vi "Process Pupil or Cornea ReflectionPerc.vi"(0 "Image In":T1, 1 "ROI":i32[](array[numeric]), 3 "Threshold":u8=130, 4 "Direction to keep":enum16{"Above", "Below"}(ring)=enum."Below", 5 "error in (no error)":errorcluster, 6 "Display":bool, 7 "Fit type":enum16{"Circle", "Ellipse"}(ring)=enum."Ellipse", 9 "Subsampling":i32=1, 10 "Color":u32(colorbox)=16711680, 11 "use % thresh":bool, 12 "Display Overlay":bool, 13 "Points to show":enum16{"All points", "Fit points"}(ring)) -> (14 "Image out":T1, 15 "x position":dbl, 17 "y position":dbl, 18 "diameter":dbl, 19 "error out":errorcluster)   [LabVIEW 2013]
uses:
  <vilib>/vision/Image Controls.llb/IMAQ Image.ctl
  Outline/Outline.lvclass
  <vilib>/Analysis/baseanly.llb/Mean (DBL).vi
  <vilib>/vision/NI_Vision_Development_Module.lvlib
  <vilib>/Analysis/NI_AALBase.lvlib
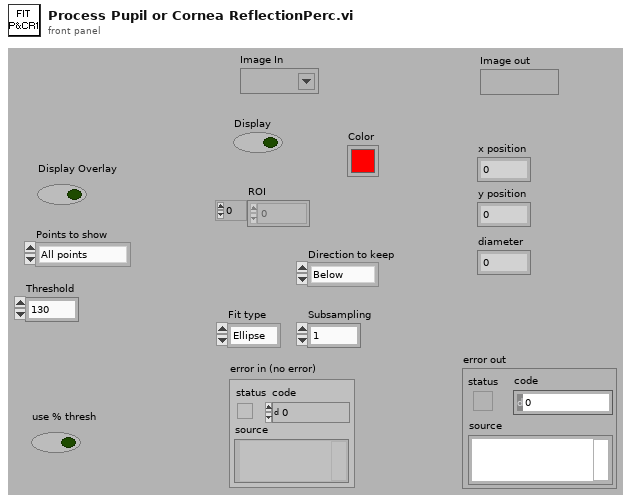
[diagram p1: front panel]
types:
  T1 = typedef "IMAQ Image.ctl" = refnum<image>
  T2 = cluster{"ROI[0]":i32, "ROI[1]":i32, "ROI[2]":i32, "ROI[3]":i32}
  T3 = cluster{"Center":cluster{"X":sgl, "Y":sgl}, "Radius":dbl}
  T4 = cluster{"Center":cluster{"X":sgl, "Y":sgl}, "Major Axis":cluster{"Point 1":cluster{"X":sgl, "Y":sgl}, "Point 2":cluster{"X":sgl, "Y":sgl}}, "Minor Axis":cluster{"Point 1":cluster{"X":sgl, "Y":sgl}, "Point 2":cluster{"X":sgl, "Y":sgl}}}
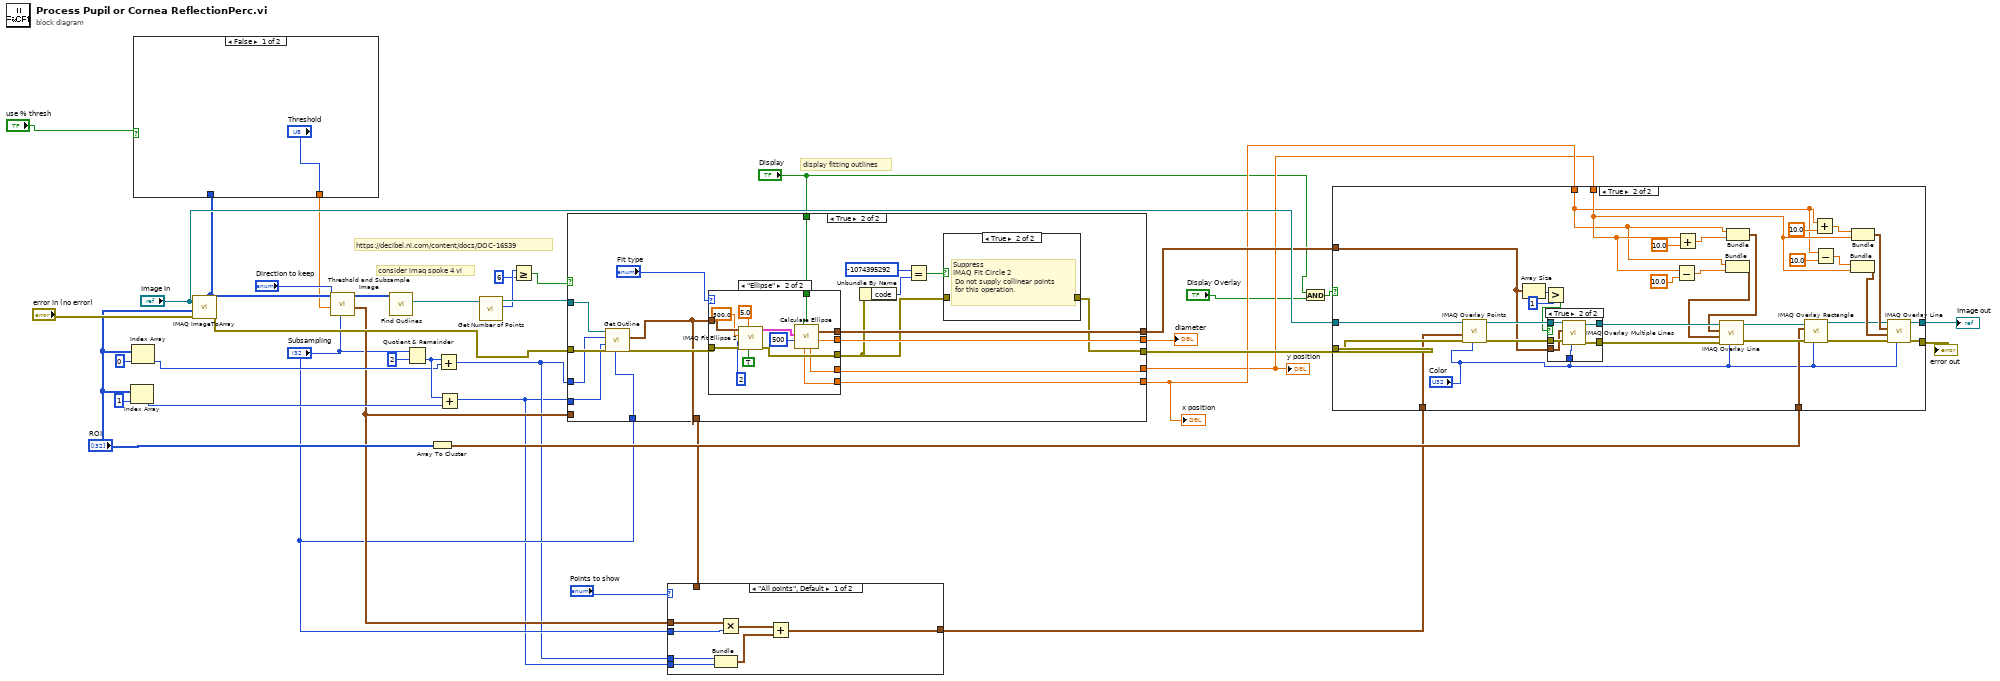
[diagram p0: block diagram]
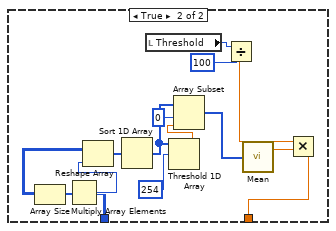
[diagram p2: hidden frame]
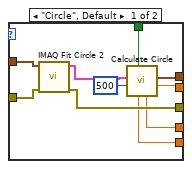
[diagram p8: hidden frame]
diagram:
  # "https://decibel.ni.com/content/docs/DOC-16539"
  # "consider imaq spoke 4 vi"
  # "display fitting outlines"
  n1 = Index Array(array="ROI", index=1) -> (element=w30:i32)
  n2 = Index Array(array="ROI", index=0) -> (element=w33:i32)
  n3 = call "IMAQ ImageToArray"("error in (no error)"="error in (no error)", "Optional Rectangle"="ROI", "Image"="Image In") -> ("error out"=w24:errorcluster, "Image Pixels (U8)"=w3:u8[][])  [unwired: 1 in, 3 out]
  n4 = case shown="False" "use % thresh" {
    tunnel: w3 -> [_ w51]
    tunnel: ["Threshold" w49] -> w1
    frame False {
    }
    frame True {
      n5 = Array Size(array=w51) -> (size(s)=w52:i32[])
      n6 = Multiply Array Elements(1:w52) -> (0:w53:i32)
      n7 = Reshape Array(w51, w53) -> (w45:u8[])
      n8 = Sort 1D Array(array=w45) -> (sorted array=w43:u8[])
      n9 = local read "Threshold"() -> (w48:u8)
      n10 = Threshold 1D Array(2:i16 254 ("threshold y"), 3:w43) -> (0:w42:dbl)  [unwired: 1 in]
      n11 = Array Subset(array=w43, index=0, length=w42) -> (w40:u8[])
      n12 = Divide(x=w48, y=u8 100) -> (x/y=w47:dbl)
      n13 = call-poly <vilib>:"Mean.vi"("X"=w40) -> ("mean"=w50:dbl)  [unwired: 1 out]
      n14 = Multiply(x=w47, y=w50) -> (x*y=w49:dbl)
    }
  }
  n15 = call "Threshold and Subsample Image.vi"("Subsample"="Subsampling", "Threshold"=w1, "Direction to keep"="Direction to keep", "Image Pixels (U8)"=w3) -> ("Cross Threshold Points"=w12:cluster{"X":i32, "Y":i32}[], "Image Pixels (U8) out"=w37:u8[][])  [unwired: 6 in]
  n16 = call "Find Outlines.vi"("Image Pixels (U8)"=w37) -> ("Largest Outline"=w25:refnum<class "Outline.lvclass">)  [unwired: 9 in, 1 out]
  n17 = Quotient & Remainder(x="Subsampling", y=2) -> (floor(x/y)=w35:i32)  [unwired: 1 out]
  n18 = Array To Cluster(array="ROI") -> (cluster=w20:T2)
  n19 = Add(x=w35, y=w33) -> (x+y=w9:i32)
  n20 = Add(x=w35, y=w30) -> (x+y=w8:i32)
  n21 = call-dynamic "Get Number of Points.vi"("Outline in"=w25) -> ("Number of points"=w28:i32, "Outline out"=w29:refnum<class "Outline.lvclass">)  [unwired: 8 in, 1 out]
  n22 = Greater Or Equal?(x=w28, y=6) -> (x >= y?=w26:bool)
  n23 = case shown="True" w26 {
    tunnel: w24 -> [w54 w72]
    tunnel: [w54 w60] -> w23
    tunnel: w9 -> [_ w57]
    tunnel: w8 -> [_ w56]
    tunnel: w29 -> [_ w71]
    tunnel: "Subsampling" -> [_ w58]
    tunnel: [_ w69] -> w19
    tunnel: [_ w67] -> w18
    tunnel: [_ w66] -> w17
    tunnel: [_ w65] -> w14
    tunnel: "Display" -> [_ w59]
    tunnel: w12 -> [_ _]
    tunnel: [_ w55] -> w13
    frame False {
    }
    frame True {
      n24 = call-dynamic "Get Outline.vi"("Scale Factor"=w58, "error in (no error)"=w72, "Y Offset"=w56, "X Offset"=w57, "Outline in"=w71) -> ("error out"=w68:errorcluster, "Outline"=w55:cluster{"X":i32, "Y":i32}[])  [unwired: 4 in, 1 out]
      n25 = case shown="\"Ellipse\"" "Fit type" {
        tunnel: w68 -> [w82 w97]
        tunnel: w55 -> [w83 w96]
        tunnel: [w81 w95] -> w61
        tunnel: [w79 w93] -> w69
        tunnel: [w78 w88] -> w67
        tunnel: [w77 w87] -> w66
        tunnel: [w75 w85] -> w65
        tunnel: w59 -> [w74 w84]
        frame "Circle", Default {
          n26 = call "IMAQ Fit Circle 2"("error in (no error)"=w82, "Radial Points"=w83) -> ("error out"=w81:errorcluster, "Circle"=w80:T3)  [unwired: 4 in, 4 out]
          n27 = call "Calculate Circle.vi"("Display"=w74, "steps"=500, "Circle"=w80) -> ("Diameter"=w75:dbl, "Circle Coordinates"=w79:cluster{"X":i32, "Y":i32}[], "y position"=w77:dbl, "x position"=w78:dbl)  [unwired: 5 in]
        }
        frame "Ellipse" {
          n28 = call "IMAQ Fit Ellipse 2"("Reject Outliers (FALSE)"=TRUE, "Pixel Radius"=5.0, "error in (no error)"=w97, "Maximum Iterations"=2, "Minimum Score"=500.0, "Radial Points"=w96) -> ("error out"=w95:errorcluster, "Ellipse"=w92:T4)  [unwired: 4 out]
          n29 = call "Calculate Ellipse.vi"("Display"=w84, "steps"=500, "Ellipse"=w92) -> ("Effective Diameter"=w85:sgl, "Ellipse Coordinates"=w93:cluster{"X":i32, "Y":i32}[], "y position"=w87:dbl, "x position"=w88:dbl)  [unwired: 5 in]
        }
      }
      n30 = Unbundle By Name(w61) -> ("code"=w64:i32)
      n31 = Equal?(x=-1074395292, y=w64) -> (x = y?=w62:bool)
      n32 = case shown="True" w62 {
        tunnel: w61 -> [w73 _]
        tunnel: [w73 _] -> w60
        frame False {
        }
        frame True {
          # "Suppress\nIMAQ Fit Circle 2\n Do not supply collinear points\n for this operation."
        }
      }
    }
  }
  "diameter" <- w14
  "x position" <- w18
  "y position" <- w17
  n33 = case shown="\"All points\", Default" "Points to show" {
    tunnel: w12 -> [w102 _]
    tunnel: "Subsampling" -> [w101 _]
    tunnel: w9 -> [w100 _]
    tunnel: w8 -> [w99 _]
    tunnel: [w98 w105] -> w7
    tunnel: w13 -> [_ w105]
    frame "All points", Default {
      n34 = Bundle(w100, w99) -> (w104:cluster{i32, i32})  [unwired: 1 in]
      n35 = Multiply(x=w102, y=w101) -> (x*y=w103:cluster{"X":i32, "Y":i32}[])
      n36 = Add(x=w103, y=w104) -> (x+y=w98:cluster{i32, i32}[])
    }
    frame "Fit points" {
    }
  }
  n37 = And(x="Display", y="Display Overlay") -> (x .and. y?=w4:bool)
  n38 = case shown="True" w4 {
    tunnel: w23 -> [w107 w111]
    tunnel: "Image In" -> [w106 w110]
    tunnel: w19 -> [_ w135]
    tunnel: [w107 w124] -> w16
    tunnel: w18 -> [_ w120]
    tunnel: w17 -> [_ w123]
    tunnel: w20 -> [_ w113]
    tunnel: [w106 w112] -> w15
    tunnel: w7 -> [_ w108]
    frame False {
    }
    frame True {
      n39 = call "IMAQ Overlay Points"("Color"="Color", "error in (no error)"=w111, "Array of Points"=w108, "Image"=w110) -> ("error out"=w139:errorcluster, "Image Out"=w140:T1)  [unwired: 6 in]
      n40 = Array Size(array=w135) -> (size(s)=w138:i32)
      n41 = Greater?(x=w138, y=1) -> (0:w136:bool)
      n42 = case shown="True" w136 {
        tunnel: w140 -> [w142 w148]
        tunnel: w139 -> [w141 w147]
        tunnel: [w142 w146] -> w133
        tunnel: [w141 w145] -> w134
        tunnel: w135 -> [_ w144]
        tunnel: "Color" -> [_ w143]
        frame False {
        }
        frame True {
          n43 = call "IMAQ Overlay Multiple Lines"("Color"=w143, "error in (no error)"=w147, "Line End Points"=w144, "Image"=w148) -> ("error out"=w145:errorcluster, "Image Out"=w146:T1)  [unwired: 6 in]
        }
      }
      n44 = Subtract(x=w123, y=10.0) -> (x-y=w128:dbl)
      n45 = Add(x=w123, y=10.0) -> (x+y=w131:dbl)
      n46 = Bundle("x position"=w120, w128) -> (w127:cluster{"x position":dbl, dbl})  [unwired: 1 in]
      n47 = Bundle("x position"=w120, w131) -> (w130:cluster{"x position":dbl, dbl})  [unwired: 1 in]
      n48 = call "IMAQ Overlay Line"("Color"="Color", "error in (no error)"=w134, "End Point"=w127, "Start Point"=w130, "Image"=w133) -> ("error out"=w114:errorcluster, "Image Out"=w117:T1)  [unwired: 5 in]
      n49 = call "IMAQ Overlay Rectangle"("Color"="Color", "error in (no error)"=w114, "Rectangle"=w113, "Image"=w117) -> ("error out"=w115:errorcluster, "Image Out"=w116:T1)  [unwired: 6 in]
      n50 = Add(x=w120, y=10.0) -> (x+y=w119:dbl)
      n51 = Subtract(x=w120, y=10.0) -> (x-y=w118:dbl)
      n52 = Bundle(w118, "y position"=w123) -> (w125:cluster{dbl, "y position":dbl})  [unwired: 1 in]
      n53 = Bundle(w119, "y position"=w123) -> (w126:cluster{dbl, "y position":dbl})  [unwired: 1 in]
      n54 = call "IMAQ Overlay Line"("Color"="Color", "error in (no error)"=w115, "End Point"=w125, "Start Point"=w126, "Image"=w116) -> ("error out"=w124:errorcluster, "Image Out"=w112:T1)  [unwired: 5 in]
    }
  }
  "error out" <- w16
  "Image out" <- w15
